vi "piezoWriteWrite.vi"(1 "mode":u16(ring) items=["fractional", "position", "voltage"], 2 "input":dbl) -> ()   [LabVIEW 2017]
uses:
  <vilib>/DAQmx/write.llb/DAQmx Write (Analog DBL 1Chan 1Samp).vi
  globalDevices.vi
  <vilib>/DAQmx/miscellaneous.llb/DAQmx Fill In Error Info.vi
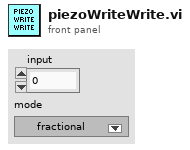
[diagram p1: front panel]
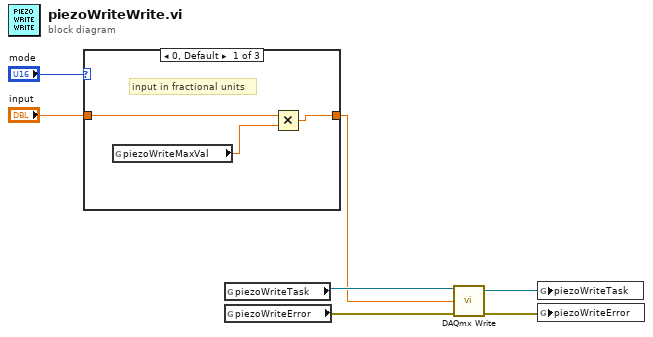
[diagram p0: block diagram]
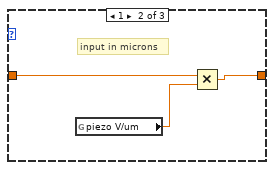
[diagram p2: hidden frame]
diagram:
  n1 = case shown="0, Default" "mode" {
    tunnel: "input" -> [w9 w13 w14]
    tunnel: [w8 w11 w14] -> w3
    frame 0, Default {
      # "input in fractional units"
      n2 = global read "globalDevices.vi" "piezoWriteMaxVal"() -> (w10:dbl)
      n3 = Multiply(x=w9, y=w10) -> (x*y=w8:dbl)
    }
    frame 1 {
      # "input in microns"
      n4 = global read "globalDevices.vi" "piezo V/um"() -> (w12:dbl)
      n5 = Multiply(x=w13, y=w12) -> (x*y=w11:dbl)
    }
    frame 2 {
      # "input in volts"
    }
  }
  n6 = global read "globalDevices.vi" "piezoWriteTask"() -> (w7:refnum<k21>)
  n7 = global read "globalDevices.vi" "piezoWriteError"() -> (w6:errorcluster)
  n8 = call-poly <vilib>:"DAQmx Write.vi"("task/channels in"=w7, "data"=w3, "error in"=w6) -> ("task out"=w2:refnum<k21>, "error out"=w1:errorcluster)  [unwired: 10 in, 1 out]
  n9 = global write "globalDevices.vi" "piezoWriteTask"(w2) -> ()
  n10 = global write "globalDevices.vi" "piezoWriteError"(w1) -> ()
